vi "ModuleManager Compile.vi"(8 "error in":errorcluster, 11 "Section Ref in":T1 format="%.0x") -> (0 "error out":errorcluster, 1 "SensorInfos":T2, 2 "Channel Refs":T1[](array[typedef]) format="%.0x", 3 "Section Ref out":T1 format="%.0x")   [LabVIEW 2023, in "Vires VTD System Explorer.lvlib"]
uses:
  Vires VTD System Explorer.lvlib
  <vilib>/NI VeriStand/Custom Device API/Custom Device Item Ref.ctl
  Shared/SensorInfos.ctl
  Shared/SensorInfo.ctl
  Shared/Sensor Name.ctl
  Shared/Protocol.ctl
  MM/MM Data.ctl
  MM/MM Objects.ctl
  MM/MM Object.ctl
  <vilib>/NI VeriStand/Custom Device Tools/Custom Device Utility Library/NI VeriStand - Search for Item by Name.vi
  <vilib>/NI VeriStand/Custom Device API/Get Item Property (Variant).vi
  <vilib>/NI VeriStand/Custom Device API/Custom Device API.lvlib
  <vilib>/NI VeriStand/Custom Device Tools/Custom Device Utility Library/Custom Device Utility Library.lvlib
  Shared/Vires VTD Shared.lvlib
  MM/MM.lvlib
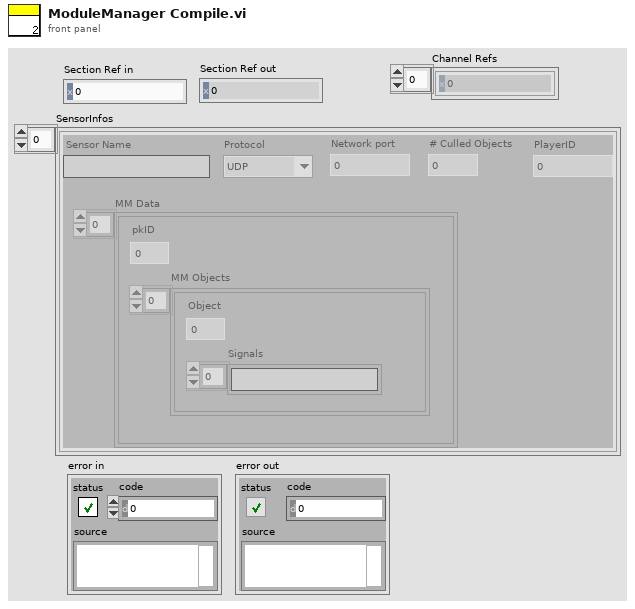
[diagram p1: front panel]
types:
  T1 = typedef "Custom Device API.lvlib/Custom Device Item Ref.ctl" = u64
  T2 = typedef "Vires VTD Shared.lvlib/SensorInfos.ctl" = T3[]
  T3 = typedef "Vires VTD Shared.lvlib/SensorInfo.ctl" = cluster{"Sensor Name":T4, "Protocol":T5, "Network port":i32, "# Culled Objects":i32, "PlayerID":u8, "MM Data":T6}
  T4 = typedef "Vires VTD Shared.lvlib/Sensor Name.ctl" = string
  T5 = typedef "Vires VTD Shared.lvlib/Protocol.ctl" = enum16{"UDP", "TCP"}
  T6 = typedef "Vires VTD Shared.lvlib/MM Data.ctl" = T7[]
  T7 = typedef "MM.lvlib/MM Objects.ctl" = cluster{"pkID":i32, "MM Objects":T8[]}
  T8 = typedef "MM.lvlib/MM Object.ctl" = cluster{"Object":i32, "Signals":string[]}
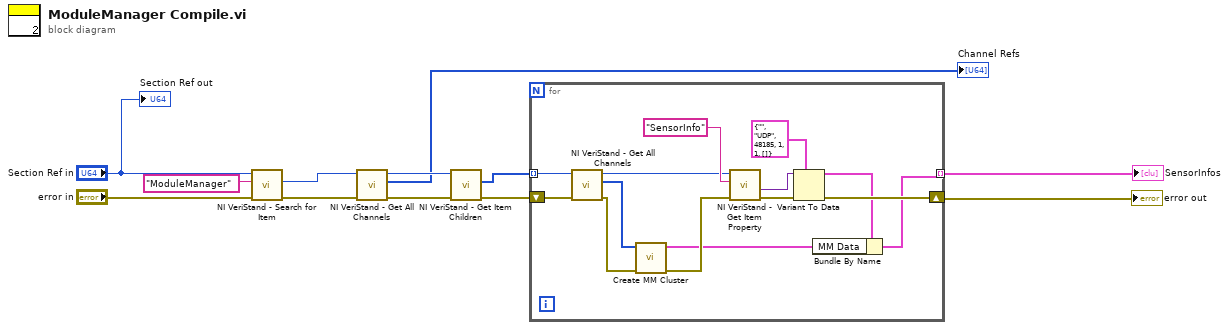
[diagram p0: block diagram]
diagram:
  n1 = call-poly <vilib>:"NI VeriStand - Search for Item.vi"("error in"="error in", "Item Name"="ModuleManager", "Section Ref in"="Section Ref in") -> ("error out"=w8:errorcluster, "Item Ref"=w6:T1)  [unwired: 5 in, 2 out]
  n2 = call <vilib>:"NI VeriStand - Get All Channels.vi"("error in"=w8, "Section Ref in"=w6) -> ("error out"=w7:errorcluster, "Channel Refs"=→"Channel Refs":T1[], "Section Ref out"=w5:T1)  [unwired: 6 in, 1 out]
  n3 = call <vilib>:"NI VeriStand - Get Item Children.vi"("error in (no error)"=w7, "Item Ref in"=w5) -> ("error out"=w9:errorcluster, "Child Refs"=w2:T1[])  [unwired: 6 in, 2 out]
  n4 = for {
    tunnel: w2 -> [w14] mode=indexing
    shift-right: [w26] -> w4
    shift-left: w9 -> [w21]
    tunnel: [w13] -> w1 mode=indexing
    n5 = call <vilib>:"NI VeriStand - Get All Channels.vi"("error in"=w21, "Section Ref in"=w14) -> ("error out"=w18:errorcluster, "Channel Refs"=w17:T1[], "Section Ref out"=w20:T1)  [unwired: 6 in, 1 out]
    n6 = call "Create MM Cluster.vi"("error out"=w18, "Channel Refs"=w17) -> ("error out 2"=w16:errorcluster, "MM Data"=w15:T6)  [unwired: 8 in]
    n7 = call-poly <vilib>:"NI VeriStand - Get Item Property.vi"("error in (no error)"=w16, "Property Name"="SensorInfo", "Item Ref in"=w20) -> ("error out"=w25:errorcluster, "Value"=w24:variant)  [unwired: 5 in, 2 out]
    n8 = Variant To Data(error in=w25, type=T3 {"Sensor Name"="", "Protocol"=enum."UDP", "Network port"=48185, "# Culled Objects"=1, "PlayerID"=1, "MM Data"=[]} ("SensorInfo"), Variant=w24) -> (data=w19:T3, error out=w26:errorcluster)
    n9 = Bundle By Name(cluster=w19, "MM Data"=w15) -> (w13:T3)
  }
  "error out" <- w4
  "SensorInfos" <- w1
  "Section Ref out" <- "Section Ref in"
